vi "Get U8 Data.vi"(7 "Subgroup":string, 8 "error in":errorcluster, 9 "Variable":string, 10 "Group":string, 11 "CVT Session In":T1) -> (0 "error out":errorcluster, 1 "found":bool, 2 "U8":u8, 3 "CVT Session Out":T1)   [LabVIEW 2014, in "CVT.lvclass"]
uses:
  CVT.lvclass
  <userlib>/_Session Fwk/Typedefs/Session Handle.ctl
  <userlib>/_Session Fwk/Session - Root.lvclass
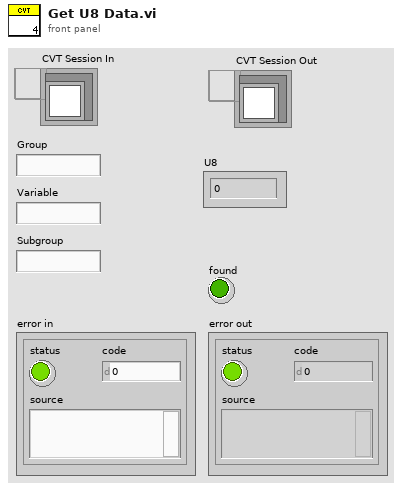
[diagram p1: front panel]
types:
  T1 = typedef "Session - Root.lvclass/Session Handle.ctl" = refnum<data-value>
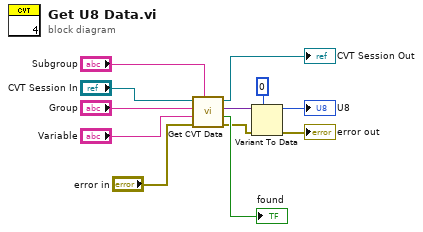
[diagram p0: block diagram]
diagram:
  n1 = call "Get CVT Data.vi"("Subgroup"="Subgroup", "error in"="error in", "Variable"="Variable", "Group"="Group", "CVT Session In"="CVT Session In") -> ("error out"=w4:errorcluster, "found"=→"found":bool, "Data Out"=w5:variant, "CVT Session Out"=→"CVT Session Out":T1)  [unwired: 3 in]
  n2 = Variant To Data(error in=w4, type=u8 0, Variant=w5) -> (data=→"U8":u8, error out=→"error out":errorcluster)
